vi "test_has_mapping.vi"() -> ()   [LabVIEW 2022 SP3]
uses:
  5ce22b75-73c9-4682-9706-e24cc5b6ee6e.vi
  yaq_labview/yaq_labview_error_handler.vi
  <vilib>/Utility/error.llb/Simple Error Handler.vi
panel:
  out "mapping ID":dbl
  out "units":string
  out "Map Out":dbl[](array[numeric])
  out "Channel Names Out":string[](array[string])
  in  "Python path":path=path "C:/ProgramData/Anaconda3/envs/lv4/pythonw.exe"
  in  "Python version":string="3.8.0"
  in  "Python Module Path":path=path "C:/Users/kamey/work/labview/yaqc-labview/python/yaqc_labview.py"
  in  "Port":i32=39004
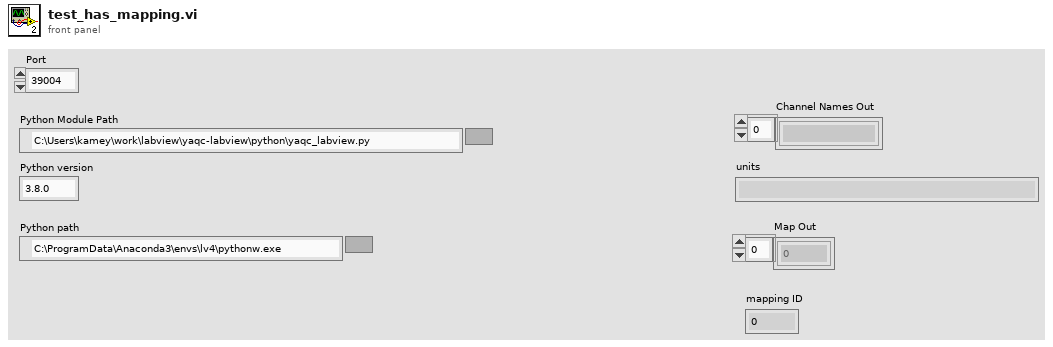
[diagram p1: front panel]
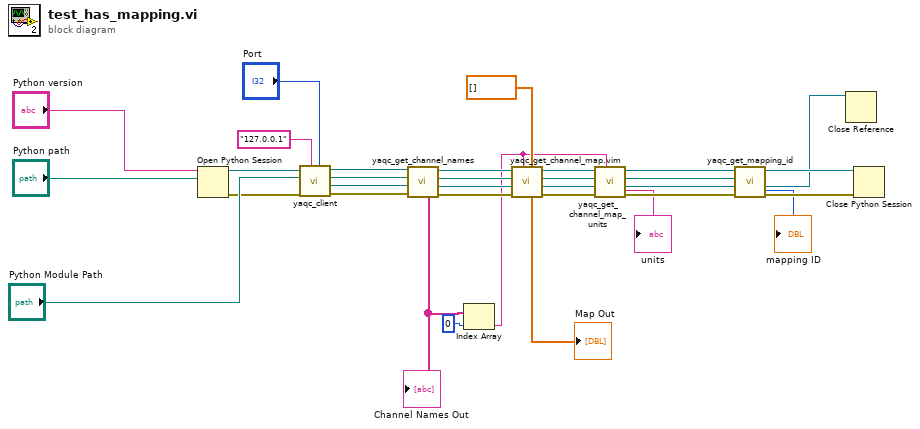
[diagram p0: block diagram]
diagram:
  n1 = Open Python Session(python version="Python version", python path="Python path") -> (session out=w28:refnum<k35>, error out=w27:errorcluster)  [unwired: 1 in]
  n2 = call "yaqc_client.vi"("Port"="Port", "host ('127.0.0.1')"="127.0.0.1", "error in (no error)"=w27, "Python Module Path"="Python Module Path", "Python Session In"=w28) -> ("error out"=w14:errorcluster, "Yaqc Client"=w3:refnum<k38>, "Python Module Path Out"=w2:path, "Python Session Out"=w1:refnum<k35>)  [unwired: 3 in]
  n3 = call "yaqc_get_channel_names.vi"("error in (no error)"=w14, "Yaqc Client In"=w3, "Python Module Path In"=w2, "Python Session In"=w1) -> ("error out"=w15:errorcluster, "Yaqc Client Out"=w13:refnum<k38>, "Python Module Path Out"=w12:path, "Python Session Out"=w11:refnum<k35>, "Channel Names Out"=w4:string[])  [unwired: 3 in]
  "Channel Names Out" <- w4
  n4 = Index Array(array=w4, index=0) -> (element=w5:string)
  n5 = call "yaqc_get_channel_map.vim"("Map In"=dbl[] [], "channel_name"=w5, "error in (no error)"=w15, "Yaqc Client In"=w13, "Python Module Path In"=w12, "Python Session In"=w11) -> ("error out"=w26:errorcluster, "Yaqc Client Out"=w21:refnum<k38>, "Python Module Path Out"=w19:path, "Python Session Out"=w17:refnum<k35>, "Map Out"=→"Map Out":dbl[])  [unwired: 1 in]
  n6 = call "yaqc_get_channel_map_units.vi"("channel_name"=w5, "error in (no error)"=w26, "Yaqc Client In"=w21, "Python Module Path In"=w19, "Python Session In"=w17) -> ("error out"=w25:errorcluster, "Yaqc Client Out"=w20:refnum<k38>, "Python Module Path Out"=w18:path, "Python Session Out"=w16:refnum<k35>, "units"=→"units":string)  [unwired: 2 in]
  n7 = call "yaqc_get_mapping_id.vi"("error in (no error)"=w25, "Yaqc Client In"=w20, "Python Module Path In"=w18, "Python Session In"=w16) -> ("error out"=w24:errorcluster, "Yaqc Client Out"=w22:refnum<k38>, "Python Session Out"=w23:refnum<k35>, "mapping ID"=→"mapping ID":i32)  [unwired: 3 in, 1 out]
  n8 = Close Reference(reference=w22) -> ()  [unwired: 1 in, 1 out]
  n9 = Close Python Session(session in=w23, error in=w24) -> ()  [unwired: 1 out]
